vi "PDLM_CreateSupportRequestText.vi"(6 "Options":u32, 8 "error in (no error)":errorcluster, 9 "CallingSW":string, 10 "Preamble":string, 11 "USBIdx":i32) -> (0 "error out":errorcluster, 2 "Buffer":string, 3 "return type":i32)   [LabVIEW 2017]
uses:
  PDLM_DllPath_global.vi
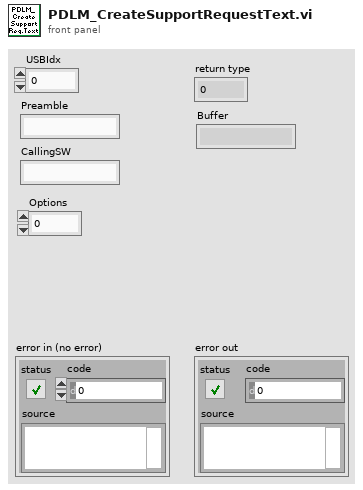
[diagram p1: front panel]
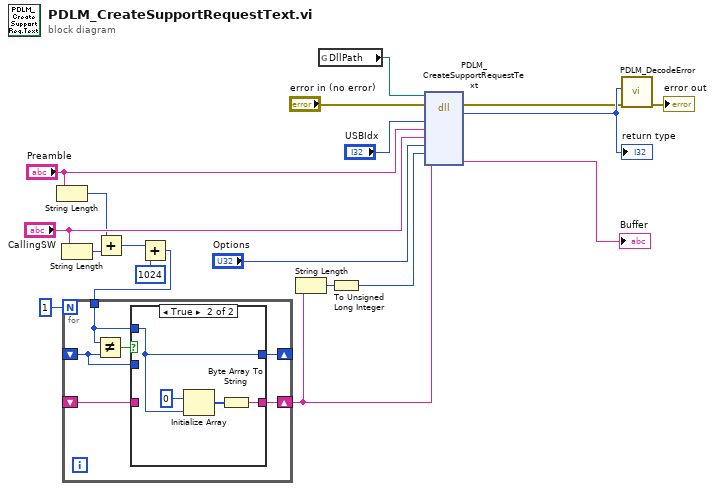
[diagram p0: block diagram]
diagram:
  n1 = String Length(string="Preamble") -> (length=w5:i32)
  n2 = String Length(string="CallingSW") -> (length=w4:i32)
  n3 = Add(x=w5, y=w4) -> (x+y=w3:i32)
  n4 = Add(x=w3, y=1024) -> (x+y=w1:i32)
  n5 = for {
    N: 1 -> [_]
    shift-right: [w25] -> w8
    shift-left: _ -> [w24]
    shift-right: [w21] -> _
    shift-left: _ -> [w20]
    tunnel: w1 -> [w22]
    n6 = Not Equal?(x=w22, y=w20) -> (x != y?=w23:bool)
    n7 = case shown="True" w23 {
      tunnel: [w27 w29] -> w25
      tunnel: w24 -> [w27 _]
      tunnel: w22 -> [_ w28]
      tunnel: [w26 w28] -> w21
      tunnel: w20 -> [w26 _]
      frame False {
      }
      frame True {
        n8 = Initialize Array(u8 0, w28) -> (w30:u8[])
        n9 = Byte Array To String(unsigned byte array=w30) -> (string=w29:string)
      }
    }
  }
  n10 = String Length(string=w8) -> (length=w13:i32)
  n11 = global read "PDLM_DllPath_global.vi" "DllPath"() -> (w15:path)
  n12 = To Unsigned Long Integer(number=w13) -> (unsigned 32bit integer=w11:u32)
  n13 = dll-call lib="M:/_dev/progs/LabVIEW/_lib/PQ/Taiko/pdlm_lib.dll" fn="PDLM_CreateSupportRequestText"(path in=w15, error in="error in (no error)", "USBIdx"="USBIdx", "Preamble"="Preamble", "CallingSW"="CallingSW", "Options"="Options", "BuffLen"=w11, "Buffer"=w8) -> (error out=w17:errorcluster, "return type"=w18:i32, "Buffer"=→"Buffer":string)  [unwired: 6 in, 1 out]
  "return type" <- w18
  n14 = call "PDLM_DecodeError.vi"("error in (no error)"=w17, "code"=w18) -> ("error out"=→"error out":errorcluster)  [unwired: 7 in, 2 out]
